vi "svl_RC Filter Coefficients.vi"(11 "dt":dbl) -> (2 "filter coefficients":cluster{"beta":dbl, "gamma":dbl, "alpha":dbl} {"alpha" format="%.2f"; "gamma" format="%.2f"; "beta" format="%.2f"})   [LabVIEW 2017, in "SoundVib_Integration.lvlib"]
uses:
  <vilib>/addons/Sound and Vibration/svt_Integration/SoundVib_Integration.lvlib
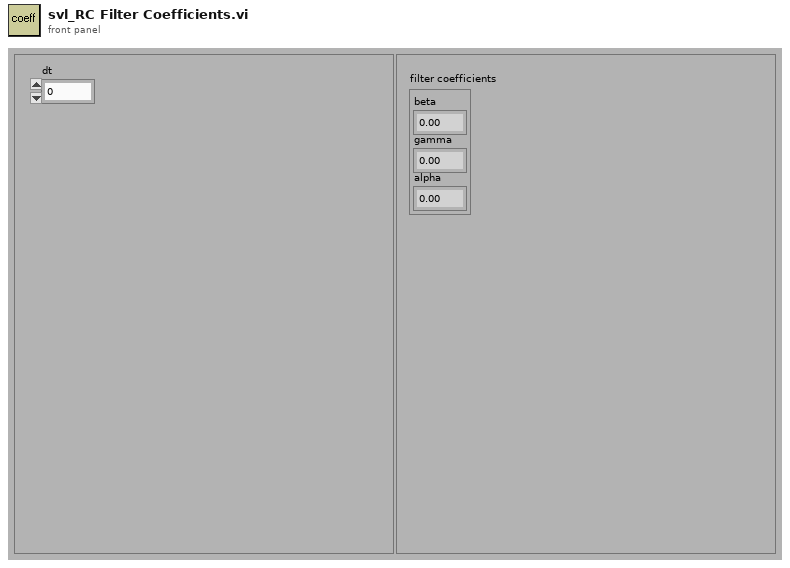
[diagram p1: front panel]
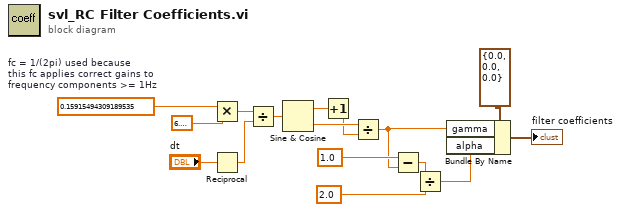
[diagram p0: block diagram]
diagram:
  w16 = 0.15915494309189535  # fc = 1/(2pi) used because  this fc applies correct gains to  frequency components >= 1Hz
  n1 = Multiply(x=w16, y=6.283185307179586) -> (x*y=w10:dbl)
  n2 = Reciprocal(x="dt") -> (1/x=w11:dbl)
  n3 = Divide(x=w10, y=w11) -> (x/y=w9:dbl)
  n4 = Sine & Cosine(0:w9) -> (1:w14:dbl, 2:w13:dbl)
  n5 = Increment(x=w14) -> (x+1=w12:dbl)
  n6 = Divide(x=w13, y=w12) -> (x/y=w4:dbl)
  n7 = Subtract(x=1.0, y=w4) -> (x-y=w7:dbl)
  n8 = Divide(x=w7, y=2.0) -> (x/y=w3:dbl)
  n9 = Bundle By Name(cluster=cluster{"beta":dbl, "gamma":dbl, "alpha":dbl} {"beta"=0.0, "gamma"=0.0, "alpha"=0.0} ("filter coefficients"), "gamma"=w4, "alpha"=w3) -> (→"filter coefficients":cluster{"beta":dbl, "gamma":dbl, "alpha":dbl})
